vi "N Teeth M Missing Page.vi"(8 "error in (no error)":errorcluster, 11 "Node Ptr":T3 format="%.0x") -> (0 "error out":errorcluster)   [LabVIEW 2011, in "Engine Sim System Explorer.lvlib"]
uses:
  Engine Sim System Explorer.lvlib
  <vilib>/NI Veristand/Custom Device API/Custom Device Item Ref.ctl
  TypeDefs/AngleReference.ctl
  TypeDefs/NTeethSettings.ctl
  Shared/Engine Simulation Global.vi
  <vilib>/NI Veristand/Custom Device API/Get Item Property (Boolean).vi
  <vilib>/NI Veristand/Custom Device API/Get Item Property (Variant).vi
  <vilib>/NI Veristand/Custom Device API/Set Item Property (Variant).vi
  <vilib>/NI Veristand/Custom Device API/Set Item Property (Boolean).vi
  <vilib>/NI Veristand/Custom Device API/Custom Device API.lvlib
  Engine Simulation Shared.lvlib
panel:
  in  "CycleAngle?":T1 caption="FPGA Simulation Angle Reference"
  in  "SHDocVw.IWebBrowser2":refnum<k7>(container)
  out "N Teeth M Missing View":picture
  in  "TDC Configuration":T2(ring)
  in  "Location Missing Teeth":dbl caption="Location of Missing Teeth After TDC"
  in  "Tooth/Gap Duty Cycle":dbl
  in  "Number Missing Teeth":u8 caption="Number of Missing Teeth"
  in  "Number of Teeth":u8
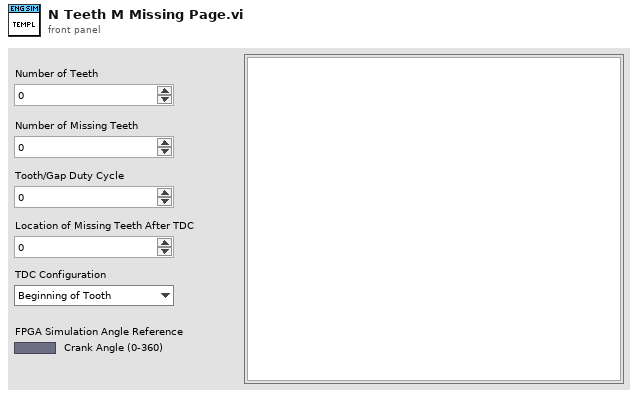
[diagram p1: front panel]
types:
  T1 = typedef "Engine Sim System Explorer.lvlib/AngleReference.ctl" = bool
  T2 = enum16{"Beginning of Tooth", "Middle of Tooth", "Beginning of Gap", "Middle of Gap"}
  T3 = typedef "Custom Device API.lvlib/Custom Device Item Ref.ctl" = u64
  T4 = typedef "Engine Sim System Explorer.lvlib/NTeethSettings.ctl" = cluster{"Tooth/Gap Duty Cycle":dbl, "Number of Teeth":u8, "Number Missing Teeth":u8, "Location Missing Teeth":dbl, "TDC Configuration":enum16{"Beginning of Tooth", "Middle of Tooth", "Beginning of Gap", "Middle of Gap"}}
  T5 = typedef "Custom Device API.lvlib/Custom Device Commands.ctl" = enum16{"Default", "Item renamed", "Shutdown", "Dynamic button pressed"}
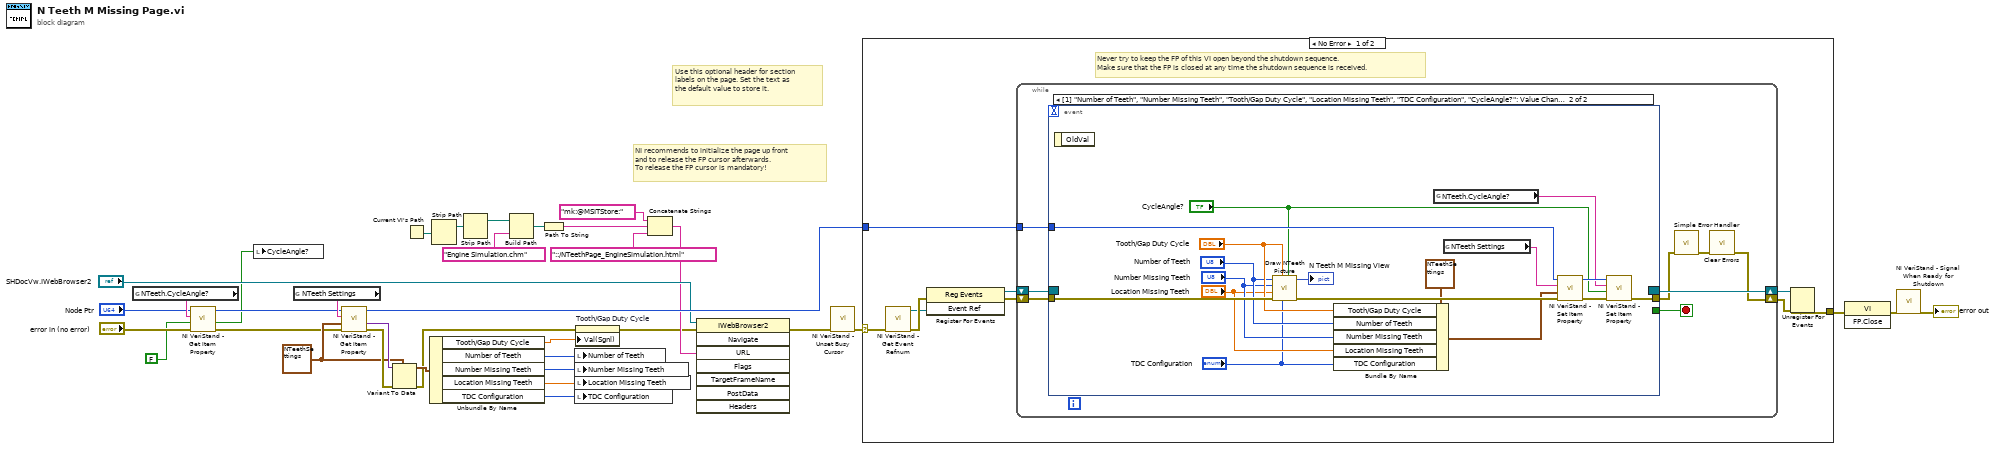
[diagram p0: block diagram]
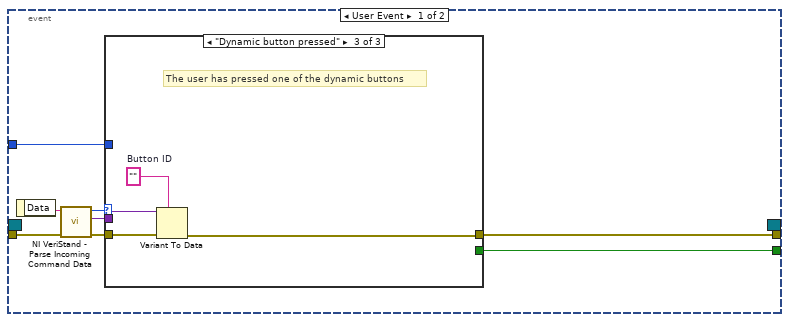
[diagram p2: hidden frame]
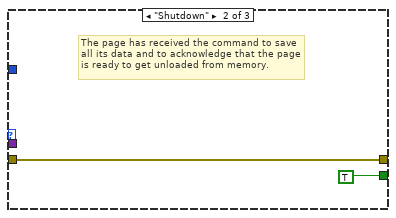
[diagram p4: hidden frame]
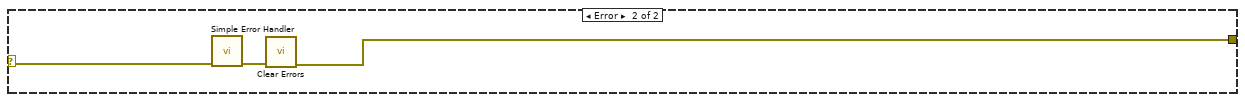
[diagram p5: hidden frame]
diagram:
  w15 = T4 {"Tooth/Gap Duty Cycle"=50.0, "Number of Teeth"=60, "Number Missing Teeth"=2, "Location Missing Teeth"=300.0, "TDC Configuration"=enum."Beginning of Tooth"} ("output cluster")
  # "Use this optional header for section labels on the page. Set the text as the default value to store it."
  # "NI recommends to initialize the page up front\nand to release the FP cursor afterwards.\nTo release the FP cursor is mandatory!"
  n1 = global read "Engine Simulation Global.vi" "NTeeth.CycleAngle?"() -> (w7:string)
  n2 = call-poly <vilib>:"NI VeriStand - Get Item Property.vi"("error in (no error)"="error in (no error)", "Default Value"=FALSE, "Property Name"=w7, "Item Ref in"="Node Ptr") -> ("error out"=w4:errorcluster, "Value"=w1:bool, "Item Ref out"=w5:T3)  [unwired: 4 in, 1 out]
  n3 = local write "CycleAngle?"(w1) -> ()
  n4 = global read "Engine Simulation Global.vi" "NTeeth Settings"() -> (w19:string)
  n5 = call-poly <vilib>:"NI VeriStand - Get Item Property.vi"("error in (no error)"=w4, "Default Value"=w15, "Property Name"=w19, "Item Ref in"=w5) -> ("error out"=w17:errorcluster, "Value"=w18:variant, "Item Ref out"=w30:T3)  [unwired: 4 in, 1 out]
  n6 = Variant To Data(error in=w17, type=w15, Variant=w18) -> (data=w16:T4, error out=w10:errorcluster)
  n7 = Current VI's Path() -> (path=w22:path)
  n8 = Unbundle By Name(w16) -> ("Tooth/Gap Duty Cycle"=w8:dbl, "Number of Teeth"=w14:u8, "Number Missing Teeth"=w13:u8, "Location Missing Teeth"=w12:dbl, "TDC Configuration"=w11:T2)
  n9 = Strip Path(path=w22) -> (stripped path=w23:path)  [unwired: 1 out]
  n10 = Strip Path(path=w23) -> (stripped path=w28:path)  [unwired: 1 out]
  n11 = Build Path(base path=w28, name or relative path="Engine Simulation.chm") -> (appended path=w26:path)
  n12 = Path To String(path=w26) -> (string=w25:string)
  n13 = local write "Number of Teeth"(w14) -> ()
  n14 = local write "Number Missing Teeth"(w13) -> ()
  n15 = local write "Location Missing Teeth"(w12) -> ()
  n16 = local write "TDC Configuration"(w11) -> ()
  n17 = property on="Tooth/Gap Duty Cycle" class="DigNum (strict)"(error in=w10, "Val(Sgnl)"=w8) -> (error out=w9:errorcluster)  [unwired: 1 in, 1 out]
  n18 = Concatenate Strings("mk:@MSITStore:" ("string"), w25, "::/NTeethPage_EngineSimulation.html" ("name or relative path")) -> (w20:string)
  n19 = invoke class="IWebBrowser2" method="Navigate"(reference="SHDocVw.IWebBrowser2", error in=w9, "URL"=w20) -> (error out=w32:errorcluster)  [unwired: 5 in, 7 out]
  n20 = call <vilib>:"NI VeriStand - Unset Busy Cursor.vi"("error in (no error)"=w32) -> ("error out"=w31:errorcluster)  [unwired: 10 out]
  n21 = case shown="No Error" w31 {
    selector: w31 -> [w36 w87]
    tunnel: [w41 w85] -> w35
    tunnel: w30 -> [w37 _]
    frame No Error {
      # "Never try to keep the FP of this VI open beyond the shutdown sequence.\nMake sure that the FP is closed at any time the shutdown sequence is received."
      n22 = call <vilib>:"NI VeriStand - Get Event Refnum.vi"("error in (no error)"=w36) -> ("error out"=w44:errorcluster, "Event Ref"=w40:refnum<user-event>)  [unwired: 9 out]
      n23 = register-events(error in=w44, w40) -> (reference out=w38:refnum<event-registration>, error out=w39:errorcluster)  [unwired: 1 in]
      n24 = while {
        tunnel: w37 -> [w48]
        shift-right: [w45] -> w42
        shift-left: w39 -> [w51]
        shift-right: [w52] -> w43
        shift-left: w38 -> [w50]
        stop <- w49 stop-if-true
        n25 = event shown="[1] \"Number of Teeth\", \"Number Missing Teeth\", \"Tooth/Gap Duty Cycle\", \"Location Missing Teeth\", \"TDC Configuration\", \"CycleAngle?\": Value Change" {
          selector: w50 -> [_ _]
          dyn-events: [_ _] -> w52
          timeout: _ -> [_ _]
          tunnel: w51 -> [w60 w83]
          tunnel: [w56 _] -> w49
          tunnel: [w55 w72] -> w47
          tunnel: w48 -> [w54 w75]
          event User Event {
            n26 = event-data() -> ("Data"=w59:string)  [unwired: 1 out]
            n27 = call <vilib>:"NI VeriStand - Parse Incoming Command Data.vi"("error in (no error)"=w60, "Incoming data"=w59) -> ("error out"=w58:errorcluster, "Outgoing data"=w53:variant, "Action"=w57:T5)  [unwired: 7 out]
            n28 = case shown="\"Dynamic button pressed\"" w57 {
              tunnel: w58 -> [w61 w62 w67]
              tunnel: [_ TRUE _] -> w56
              tunnel: [w61 w62 w64] -> w55
              tunnel: w54 -> [_ _ _]
              tunnel: w53 -> [_ _ w66]
              frame "Default", Default {
              }
              frame "Shutdown" {
                # "The page has received the command to save all its data and to acknowledge that the page is ready to get unloaded from memory."
              }
              frame "Dynamic button pressed" {
                w65 = ""  # Button ID
                # "The user has pressed one of the dynamic buttons"
                n29 = Variant To Data(error in=w67, type=w65, Variant=w66) -> (error out=w64:errorcluster)  [unwired: 1 out]
              }
            }
          }
          event "Number of Teeth", "Number Missing Teeth", "Tooth/Gap Duty Cycle", "Location Missing Teeth", "TDC Configuration": Value Change {
            n30 = event-data() -> ()  [unwired: 2 out]
            n31 = call "Draw NTeeth Picture.vi"("CycleAngle?"="CycleAngle?", "TDC Configuration"="TDC Configuration", "Tooth/Gap Duty Cycle"="Tooth/Gap Duty Cycle", "error in (no error)"=w83, "Location of Missing Teeth After TDC"="Location Missing Teeth", "Number of Missing Teeth"="Number Missing Teeth", "Number of Teeth"="Number of Teeth") -> ("error out"=w77:errorcluster, "N Teeth M Missing View"=→"N Teeth M Missing View":picture)  [unwired: 3 in]
            n32 = Bundle By Name(cluster=T4 {"Tooth/Gap Duty Cycle"=50.0, "Number of Teeth"=60, "Number Missing Teeth"=2, "Location Missing Teeth"=300.0, "TDC Configuration"=enum."Beginning of Tooth"} ("output cluster"), "Tooth/Gap Duty Cycle"="Tooth/Gap Duty Cycle", "Number of Teeth"="Number of Teeth", "Number Missing Teeth"="Number Missing Teeth", "Location Missing Teeth"="Location Missing Teeth", "TDC Configuration"="TDC Configuration") -> (w76:T4)
            n33 = global read "Engine Simulation Global.vi" "NTeeth.CycleAngle?"() -> (w69:string)
            n34 = global read "Engine Simulation Global.vi" "NTeeth Settings"() -> (w74:string)
            n35 = call-poly <vilib>:"NI VeriStand - Set Item Property.vi"("error in (no error)"=w77, "Value"=w76, "Property Name"=w74, "Item Ref in"=w75) -> ("error out"=w71:errorcluster, "Item Ref out"=w70:T3)  [unwired: 5 in, 1 out]
            n36 = call-poly <vilib>:"NI VeriStand - Set Item Property.vi"("error in (no error)"=w71, "Value"="CycleAngle?", "Property Name"=w69, "Item Ref in"=w70) -> ("error out"=w72:errorcluster)  [unwired: 5 in, 2 out]
          }
        }
        n37 = call <vilib>:"Simple Error Handler.vi"("error in (no error)"=w47) -> ("error out"=w46:errorcluster)  [unwired: 1 in, 7 out]
        n38 = call <vilib>:"Clear Errors.vi"("error in (no error)"=w46) -> ("error out"=w45:errorcluster)  [unwired: 6 out]
      }
      n39 = Unregister For Events(event registration refnum=w43, error in=w42) -> (error out=w41:errorcluster)
    }
    frame Error {
      n40 = call <vilib>:"Simple Error Handler.vi"("error in (no error)"=w87) -> ("error out"=w86:errorcluster)  [unwired: 1 in, 7 out]
      n41 = call <vilib>:"Clear Errors.vi"("error in (no error)"=w86) -> ("error out"=w85:errorcluster)  [unwired: 6 out]
    }
  }
  n42 = invoke class="VI" method="FP.Close"(error in=w35) -> (error out=w34:errorcluster)  [unwired: 2 in, 2 out]
  n43 = call <vilib>:"NI VeriStand - Signal When Ready for Shutdown.vi"("error in (no error)"=w34) -> ("error out"=→"error out":errorcluster)  [unwired: 10 out]
